vi "delete array全部的0.vi"(3 "origin":i32[][](array[numeric])) -> (0 "fin正":i32[][](array[numeric]), 1 "FIN倒":i32[][](array[numeric]))   [LabVIEW 2015]
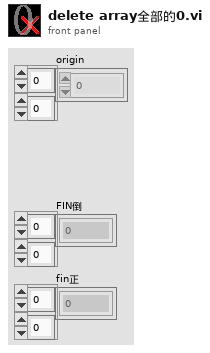
[diagram p1: front panel]
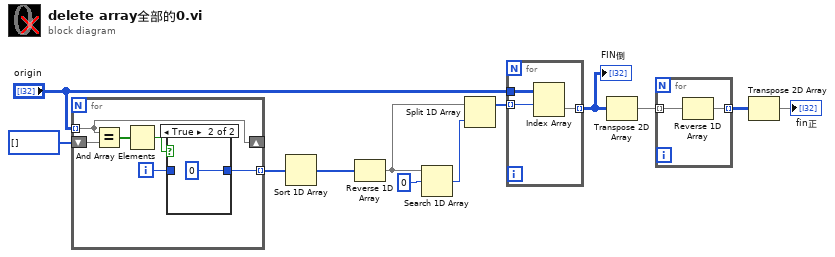
[diagram p0: block diagram]
diagram:
  n1 = for {
    tunnel: "origin" -> [w18] mode=indexing
    shift-right: [w18] -> _
    shift-left: i32[] [] ("origin") -> [w17]
    tunnel: [w13] -> w2 mode=indexing
    i -> [w14]
    n2 = Equal?(x=w18, y=w17) -> (x = y?=w16:bool[])
    n3 = And Array Elements(Boolean array=w16) -> (logical AND=w15:bool)
    n4 = case shown="True" w15 {
      tunnel: w14 -> [w19 _]
      tunnel: [w19 0] -> w13
      frame False {
      }
      frame True {
      }
    }
  }
  n5 = Sort 1D Array(array=w2) -> (sorted array=w1:i32[])
  n6 = Reverse 1D Array(array=w1) -> (reversed array=w11:i32[])
  n7 = Search 1D Array(1D array=w11, element=0) -> (index of element=w9:i32)  [unwired: 1 in]
  n8 = Split 1D Array(array=w11, index=w9) -> (first subarray=w12:i32[])  [unwired: 1 out]
  n9 = for {
    tunnel: "origin" -> [w23]
    tunnel: w12 -> [w22] mode=indexing
    tunnel: [w21] -> w7 mode=indexing
    n10 = Index Array(array=w23, index (row)=w22) -> (element=w21:i32[])  [unwired: 1 in]
  }
  "FIN倒" <- w7
  n11 = Transpose 2D Array(2D array=w7) -> (transposed array=w8:i32[][])
  n12 = for {
    tunnel: w8 -> [w25] mode=indexing
    tunnel: [w24] -> w6 mode=indexing
    n13 = Reverse 1D Array(array=w25) -> (reversed array=w24:i32[])
  }
  n14 = Transpose 2D Array(2D array=w6) -> (transposed array=→"fin正":i32[][])
